vi "Clear.vi"(8 "error in (no error)":errorcluster, 11 "Application In":refnum<class "Application.lvclass">) -> (0 "error out":errorcluster)   [LabVIEW 2020, in "Application.lvclass"]
doc: "Clears any resorces allocated during initialization for application and owned processes."
uses:
  Application.lvclass
  Application.lvclass/Application.ctl
  Process/Process.lvclass
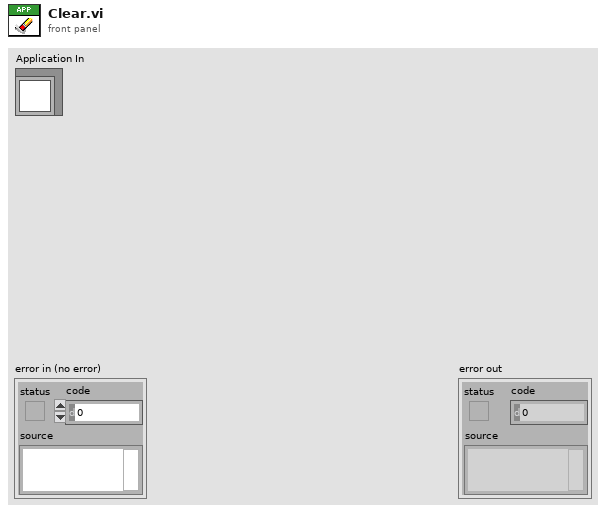
[diagram p1: front panel]
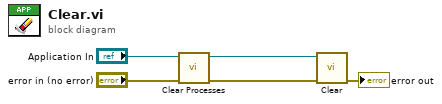
[diagram p0: block diagram]
diagram:
  n1 = call "Clear Processes.vi"("error in (no error)"="error in (no error)", "Application In"="Application In") -> ("error out"=w1:errorcluster, "Application Out"=w3:refnum<class "Application.lvclass">)  [unwired: 8 in]
  n2 = call-parent "Clear.vi"("error in (no error)"=w1, "Process In"=w3) -> ("error out"=→"error out":errorcluster)  [unwired: 9 in]
